vi "Actor Core.vi"(8 "error in":errorcluster, 11 "OD600 Actor.lvlib:OD600.lvclass":refnum<class "OD600.lvclass">) -> (0 "error out":errorcluster, 3 "Actor out":refnum<class "Actor.lvclass">)   [LabVIEW 2013, in "OD600.lvlib" / "OD600.lvclass"]
doc: "This is Actor Core.vi, the main message handling loop for Actors. An actor usually just sits in this loop and processes messages as they arrive. Any error returned by the message Do.vi call will stop the loop, with error code 43 as the canonical signal to stop with no error sent to caller. Descendants may override that in Handle Error.vi."
uses:
  OD600.lvclass
  PluginInterface/Actor Framework.lvlibp/Actor/Actor.lvclass
  OD600.lvclass/OD600.ctl
  PluginInterface/PluginInterface.lvlibp/PluginInterfaceClass/PluginInterface.lvclass
  Write Graph 1.vi
  Write Graph 2.vi
  Write Graph History.vi
  Write Growth Rate.vi
  Write Window Size.vi
  Write OD600.vi
  Write Sampling Interval.vi
  PluginInterface/PluginInterface.lvlibp/PluginInterfaceClass/Write VI Refnum.vi
  PluginInterface/Actor Framework.lvlibp/Message Enqueuer/Enqueue.vi
  OD600 Messages/Initialize Msg/Initialize Msg.lvclass
  OD600 Messages/Update Graphs Msg/Update Graphs Msg.lvclass
  OD600 Messages/Read Meter Msg/Read Meter Msg.lvclass
  OD600 Messages/Log Data Msg/Log Data Msg.lvclass
  PluginInterface/Actor Framework.lvlibp/Stop Msg/Stop Msg.lvclass
panel:
  in  "stop signal":bool
  in  "Sampling Interval":dbl=5000.0
  out "OD600":dbl
  in  "Graph History":dbl=300.0
  out "Graph 1":T1(graph) caption="Pump A"
  out "Growth Rate":dbl
  in  "Window Size":dbl=30.0
  out "Graph 2":T1(graph) caption="Pump A"
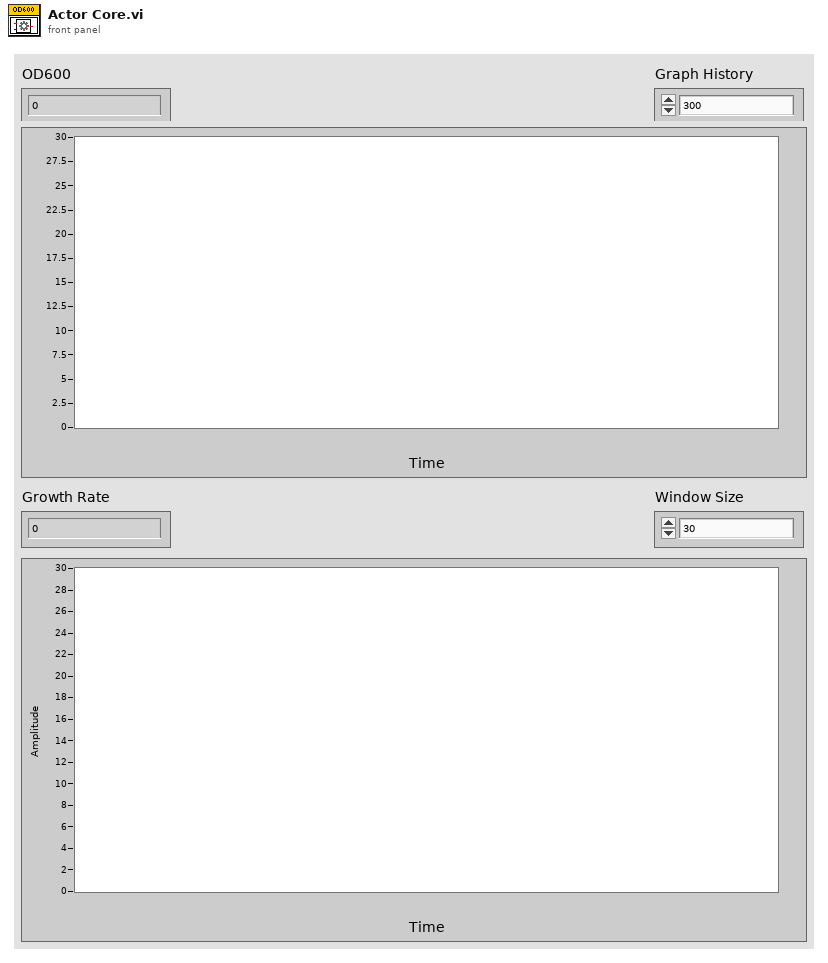
[diagram p1: front panel]
types:
  T1 = cluster{"output array":dbl[], "output array":dbl[]}
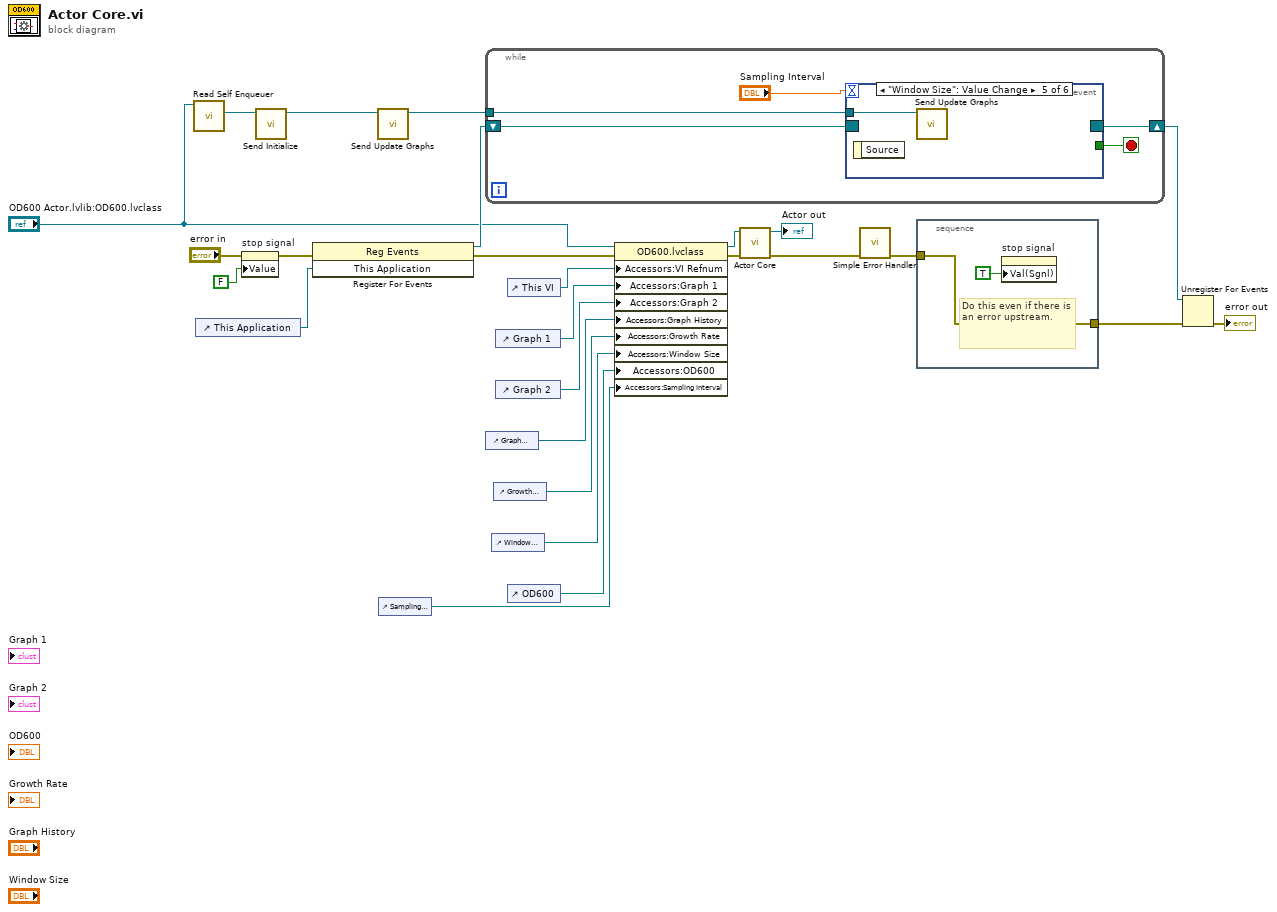
[diagram p0: block diagram]
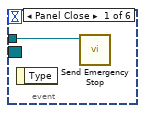
[diagram p2: hidden frame]
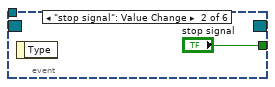
[diagram p3: hidden frame]
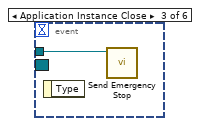
[diagram p4: hidden frame]
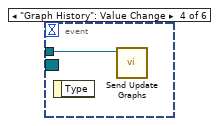
[diagram p5: hidden frame]
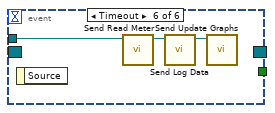
[diagram p6: hidden frame]
diagram:
  n1 = call "Read Self Enqueuer.vi"("Actor"="OD600 Actor.lvlib:OD600.lvclass") -> ("Self Enqueuer"=w7:refnum<class "Message Enqueuer.lvclass">)  [unwired: 10 in]
  n2 = control-ref of="This Application"() -> (w19:refnum<vi>)
  n3 = property on="stop signal" class="Bool (strict)"(error in="error in", "Value"=FALSE ("stop")) -> (error out=w20:errorcluster)  [unwired: 1 in, 1 out]
  n4 = call "Send Initialize.vi"("Message Enqueuer"=w7) -> ("Message Enqueuer out"=w3:refnum<class "Message Enqueuer.lvclass">)  [unwired: 9 in, 1 out]
  n5 = register-events(error in=w20, w19) -> (reference out=w23:refnum<event-registration>, error out=w4:errorcluster)  [unwired: 1 in]
  n6 = call "Send Update Graphs.vi"("Message Enqueuer"=w3) -> ("Message Enqueuer out"=w2:refnum<class "Message Enqueuer.lvclass">)  [unwired: 9 in, 1 out]
  n7 = control-ref of="Sampling Interval"() -> (w1:refnum<vi>)
  n8 = while {
    tunnel: w2 -> [w31]
    shift-right: [w29] -> w22
    shift-left: w23 -> [w28]
    stop <- w30 stop-if-true
    n9 = event shown="[4] \"Window Size\": Value Change" {
      selector: w28 -> [_ _ _ _ _ _]
      dyn-events: [_ _ _ _ _ _] -> w29
      timeout: "Sampling Interval" -> [_ _ _ _ _ _]
      tunnel: w31 -> [w32 _ w34 w35 w36 w37]
      tunnel: [_ "stop signal" _ _ _ _] -> w30
      event Panel Close {
        n10 = event-data() -> ()  [unwired: 1 in, 1 out]
        n11 = call "Send Emergency Stop.vi"("Message Enqueuer"=w32) -> ()  [unwired: 10 in, 1 out]
      }
      event "stop signal": Value Change {
        n12 = event-data() -> ()  [unwired: 1 in, 1 out]
      }
      event Application Instance Close {
        n13 = event-data() -> ()  [unwired: 1 in, 1 out]
        n14 = call "Send Emergency Stop.vi"("Message Enqueuer"=w34) -> ()  [unwired: 10 in, 1 out]
      }
      event "Graph History": Value Change {
        n15 = event-data() -> ()  [unwired: 1 in, 1 out]
        n16 = call "Send Update Graphs.vi"("Message Enqueuer"=w35) -> ()  [unwired: 9 in, 2 out]
      }
      event "Window Size": Value Change {
        n17 = event-data() -> ()  [unwired: 1 in, 1 out]
        n18 = call "Send Update Graphs.vi"("Message Enqueuer"=w36) -> ()  [unwired: 9 in, 2 out]
      }
      event Timeout {
        n19 = event-data() -> ()  [unwired: 1 in, 1 out]
        n20 = call "Send Read Meter.vi"("Message Enqueuer"=w37) -> ("Message Enqueuer out"=w38:refnum<class "Message Enqueuer.lvclass">)  [unwired: 9 in, 1 out]
        n21 = call "Send Log Data.vi"("Message Enqueuer"=w38) -> ("Message Enqueuer out"=w39:refnum<class "Message Enqueuer.lvclass">)  [unwired: 9 in, 1 out]
        n22 = call "Send Update Graphs.vi"("Message Enqueuer"=w39) -> ()  [unwired: 9 in, 2 out]
      }
    }
  }
  n23 = control-ref of="Graph History"() -> (w9:refnum<vi>)
  n24 = control-ref of="Window Size"() -> (w11:refnum<vi>)
  n25 = control-ref of="Growth Rate"() -> (w10:refnum<vi>)
  n26 = control-ref of="Graph 1"() -> (w6:refnum<vi>)
  n27 = control-ref of="Graph 2"() -> (w5:refnum<vi>)
  n28 = control-ref of="This VI"() -> (w13:refnum<vi>)
  n29 = control-ref of="OD600"() -> (w8:refnum<vi>)
  n30 = property class="OD600.lvclass"(reference="OD600 Actor.lvlib:OD600.lvclass", error in=w4, "Accessors:VI Refnum"=w13, "Accessors:Graph 1"=w6, "Accessors:Graph 2"=w5, "Accessors:Graph History"=w9, "Accessors:Growth Rate"=w10, "Accessors:Window Size"=w11, "Accessors:OD600"=w8, "Accessors:Sampling Interval"=w1) -> (reference out=w18:refnum<class "OD600.lvclass">, error out=w14:errorcluster)
  n31 = call-parent "Actor Core.vi"("error in"=w14, "Actor in"=w18) -> ("error out"=w25:errorcluster, "Actor out"=→"Actor out":refnum<class "Actor.lvclass">)  [unwired: 8 in]
  n32 = call <vilib>:"Simple Error Handler.vi"("error in (no error)"=w25) -> ("error out"=w24:errorcluster)  [unwired: 4 in, 4 out]
  n33 = stacked-sequence {
    tunnel: [w40] -> w21
    tunnel: w24 -> [w40]
    frame #0 {
      # "Do this even if there is an error upstream."
      n34 = property on="stop signal" class="Bool (strict)"("Val(Sgnl)"=TRUE ("stop")) -> ()  [unwired: 2 in, 2 out]
    }
  }
  n35 = Unregister For Events(event registration refnum=w22, error in=w21) -> (error out=→"error out":errorcluster)
